vi "SwerveDrivePoseEst2_New.vi"(4 "VisionMeasurementStdDevs":T4=[[0.9], [0.9], [0.9]], 6 "StateStdDevs":T4=[[0.1], [0.1], [0.1]], 7 "SWERVE_DRIVE_KINEMATICS":T3 {"SavedModuleStates"."Angle"."SIN" format="%13.4f"; "SavedModuleStates"."Angle"."COS" format="%13.4f"; "SavedModuleStates"."Angle"."VALUE" format="%13.4f"; "PrevCoR"."Y" format="%14.3f"; "PrevCoR"."X" format="%14.3f"; "Modules"."Y" format="%14.3f"; "Modules"."X" format="%14.3f"}, 8 "InitialPose":T7={"TRANSLATION"={"X"=0.0, "Y"=0.0}, "ROTATION"={"VALUE"=0.0, "COS"=1.0, "SIN"=0.0}} {"ROTATION"."SIN" format="%13.4f"; "ROTATION"."COS" format="%13.4f"; "ROTATION"."VALUE" format="%13.4f"; "TRANSLATION"."Y" format="%14.3f"; "TRANSLATION"."X" format="%14.3f"}, 10 "Module Positions":T1[](array[typedef]) {"Angle"."SIN" format="%13.4f"; "Angle"."COS" format="%13.4f"; "Angle"."VALUE" format="%13.4f"}, 11 "gyroAngle":T2={"VALUE"=0.0, "COS"=1.0, "SIN"=0.0} {"SIN" format="%13.4f"; "COS" format="%13.4f"; "VALUE" format="%13.4f"}) -> (0 "Error":errorcluster, 3 "SwerveDrivePoseEstimate":T8={"M_Vision_K"=[], "m_nominal_dT"=0.0, "m_PrevTime_Sec"=0.0, "Pose_Buffer"={"TimeStamps"=[], "DataArray"=[], "Min_TimeStamp"=0.0, "Max_TimeStamp"=0.0, "ItemCount"=0, "MaxBufferTime"=0.0}, "Swerve_Drive_Kinematics"={"NumModules"=0, "InverseKinematics"=[], "ForwardKinematics"=[], "Modules"=[], "PrevCoR"={"X"=0.0, "Y"=0.0}, "SavedModuleStates"=[]}, "Swerve_Drive_Odom"={"POSE"={"TRANSLATION"={"X"=0.0, "Y"=0.0}, "ROTATION"={"VALUE"=0.0, "COS"=1.0, "SIN"=0.0}}, "GyroOffset"={"VALUE"=0.0, "COS"=1.0, "SIN"=0.0}, "PreviousAngle"={"VALUE"=0.0, "COS"=1.0, "SIN"=0.0}, "PrevModulePositions"=[], "NumModules"=0}, "M_Q"=[[0.0], [0.0], [0.0]], "NumModules"=-1} {"Swerve_Drive_Odom"."PrevModulePositions"."Angle"."SIN" format="%13.4f"; "Swerve_Drive_Odom"."PrevModulePositions"."Angle"."COS" format="%13.4f"; "Swerve_Drive_Odom"."PrevModulePositions"."Angle"."VALUE" format="%13.4f"; "Swerve_Drive_Odom"."PreviousAngle"."SIN" format="%13.4f"; "Swerve_Drive_Odom"."PreviousAngle"."COS" format="%13.4f"; "Swerve_Drive_Odom"."PreviousAngle"."VALUE" format="%13.4f"; "Swerve_Drive_Odom"."GyroOffset"."SIN" format="%13.4f"; "Swerve_Drive_Odom"."GyroOffset"."COS" format="%13.4f"; "Swerve_Drive_Odom"."GyroOffset"."VALUE" format="%13.4f"; "Swerve_Drive_Odom"."POSE"."ROTATION"."SIN" format="%13.4f"; "Swerve_Drive_Odom"."POSE"."ROTATION"."COS" format="%13.4f"; "Swerve_Drive_Odom"."POSE"."ROTATION"."VALUE" format="%13.4f"; "Swerve_Drive_Odom"."POSE"."TRANSLATION"."Y" format="%14.3f"; "Swerve_Drive_Odom"."POSE"."TRANSLATION"."X" format="%14.3f"; "Swerve_Drive_Kinematics"."SavedModuleStates"."Angle"."SIN" format="%13.4f"; "Swerve_Drive_Kinematics"."SavedModuleStates"."Angle"."COS" format="%13.4f"; "Swerve_Drive_Kinematics"."SavedModuleStates"."Angle"."VALUE" format="%13.4f"; "Swerve_Drive_Kinematics"."PrevCoR"."Y" format="%14.3f"; "Swerve_Drive_Kinematics"."PrevCoR"."X" format="%14.3f"; "Swerve_Drive_Kinematics"."Modules"."Y" format="%14.3f"; "Swerve_Drive_Kinematics"."Modules"."X" format="%14.3f"})   [LabVIEW 2019, in "Trajectory_Library.lvlib"]
doc: "This class wraps Swerve Drive Odometry to fuse latency-compensated vision measurements with differential drive encoder measurements. It is intended to be a drop-in replacement for SwerveDrvOdometry; in fact, if you never call SwerveDrvPoseEst2_AddVisionMeasurement and only call SwerveDrvPoseEst2_Update then this will behave exactly the same as SwerveDrvOdometry.\n \nSwerveDrvPoseEst2_Update should be called every robot loop.\n \nSwrveDrvPoseEst2_AddVisionMeasurement can be called as infrequently as you want. If you never call it then this set of VI will behave exactly like regular encoder odometry.\n\nConstructs a SwerveDrivePoseEstimator2.\n\nThe default standard deviations of the model states are 0.1 meters for x, 0.1 meters for y, and 0.1 radians for heading. The default standard deviations of the vision measurements are 0.9 meters for x, 0.9 meters for y, and 0.9 radians for heading.\n\nInputs: \n - kinematics -- SwerveDriveKinematics -- A correctly-configured kinematics data cluster for your drivetrain.\n - gyroAngle -- Rotation2d -- The current gyro angle.\n - ModulePositions -- ModulePositions -- The current module positions.\n - initialPoseMeters -- Pose2d -- The starting pose estimate.\n - stateStdDevs -- <3,1> matrix -- Standard deviations of the pose estimate (x position in meters, y position in meters, and heading in radians). Increase these numbers to trust your state estimate less.\n - visionMeasurementStdDevs -- <3,1> matrix -- Standard deviations of the vision pose measurement (x position in meters, y position in meters, and heading in radians). Increase these numbers to trust the vision pose measurement less.\n \nOutputs:\n -- SwerveDrivePoseEst2 -- SwerveDrivePoseEst2 -- Created data cluster."
uses:
  Trajectory_Library.lvlib
  <vilib>/Analysis/Matrix/Datatypes/RealMatrix.ctl
  <vilib>/Analysis/Matrix/NI_Matrix.lvlib
  TypeDef/TRANSLATION2D.ctl
  TypeDef/ROTATION2D.ctl
  TypeDef/POSE2D.ctl
  TypeDef/TIME_INTERPOLATABLE_VARIANT.ctl
  TypeDef/SWERVE_DRIVE_MODULE_STATE.ctl
  TypeDef/SWERVE_DRIVE_KINEMATICS.ctl
  TypeDef/SWERVE_DRIVE_MODULE_POSITION.ctl
  TypeDef/SWERVE_DRIVE_ODOMETRY.ctl
  TypeDef/SWERVE_DRIVE_POSE_EST2.ctl
panel:
  # "<3,1>"
  # "<3, 1>"
  # "<3, 1>"
  # "<3, 3>"
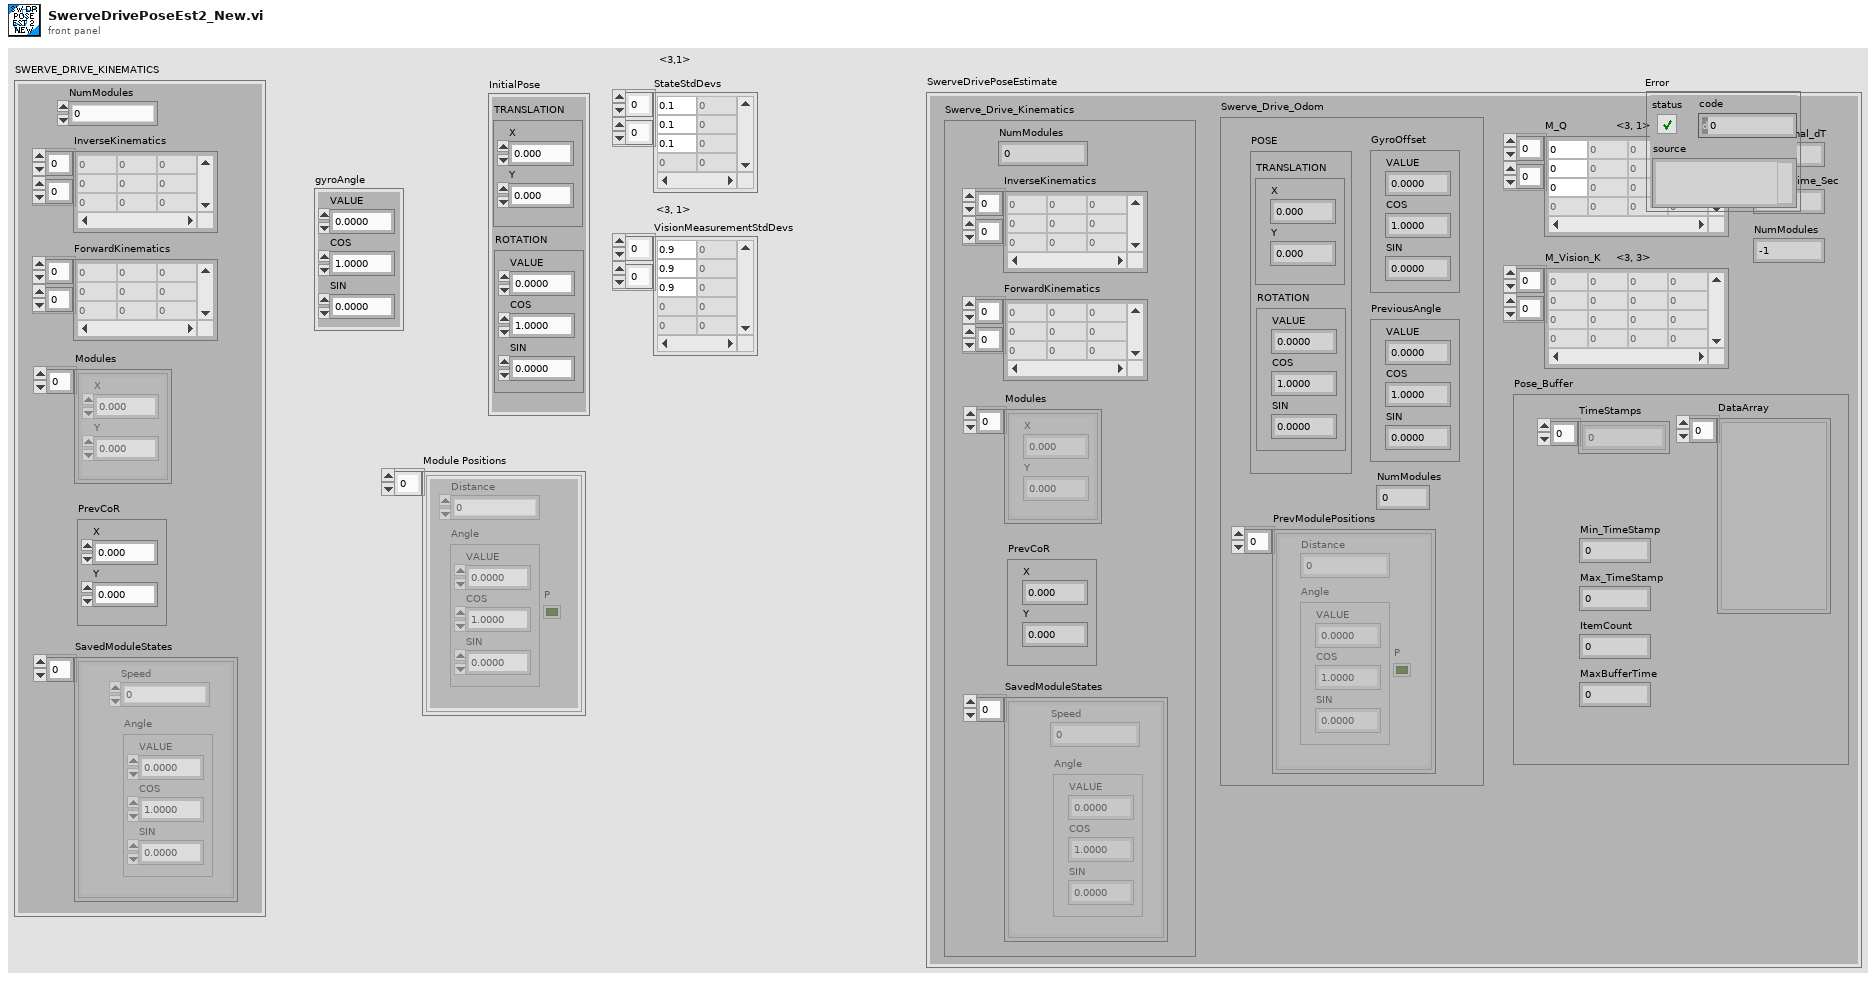
[diagram p1: front panel]
types:
  T1 = typedef "Trajectory_Library.lvlib/SWERVE_DRIVE_MODULE_POSITION.ctl" = cluster{"Distance":dbl, "Angle":T2, "P":bool}
  T2 = typedef "Trajectory_Library.lvlib/ROTATION2D.ctl" = cluster{"VALUE":dbl, "COS":dbl, "SIN":dbl}
  T3 = typedef "Trajectory_Library.lvlib/SWERVE_DRIVE_KINEMATICS.ctl" = cluster{"NumModules":i32, "InverseKinematics":T4, "ForwardKinematics":T4, "Modules":T5[], "PrevCoR":T5, "SavedModuleStates":T6[]}
  T4 = typedef "NI_Matrix.lvlib/RealMatrix.ctl" = dbl[][]
  T5 = typedef "Trajectory_Library.lvlib/TRANSLATION2D.ctl" = cluster{"X":dbl, "Y":dbl}
  T6 = typedef "Trajectory_Library.lvlib/SWERVE_DRIVE_MODULE_STATE.ctl" = cluster{"Speed":dbl, "Angle":T2}
  T7 = typedef "Trajectory_Library.lvlib/POSE2D.ctl" = cluster{"TRANSLATION":T5, "ROTATION":T2}
  T8 = typedef "Trajectory_Library.lvlib/SWERVE_DRIVE_POSE_EST2.ctl" = cluster{"M_Vision_K":T4, "m_nominal_dT":dbl, "m_PrevTime_Sec":dbl, "Pose_Buffer":T9, "Swerve_Drive_Kinematics":T3, "Swerve_Drive_Odom":T10, "M_Q":T4, "NumModules":i32}
  T9 = typedef "Trajectory_Library.lvlib/TIME_INTERPOLATABLE_VARIANT.ctl" = cluster{"TimeStamps":dbl[], "DataArray":variant[], "Min_TimeStamp":dbl, "Max_TimeStamp":dbl, "ItemCount":i32, "MaxBufferTime":dbl}
  T10 = typedef "Trajectory_Library.lvlib/SWERVE_DRIVE_ODOMETRY.ctl" = cluster{"POSE":T7, "GyroOffset":T2, "PreviousAngle":T2, "PrevModulePositions":T1[], "NumModules":i32}
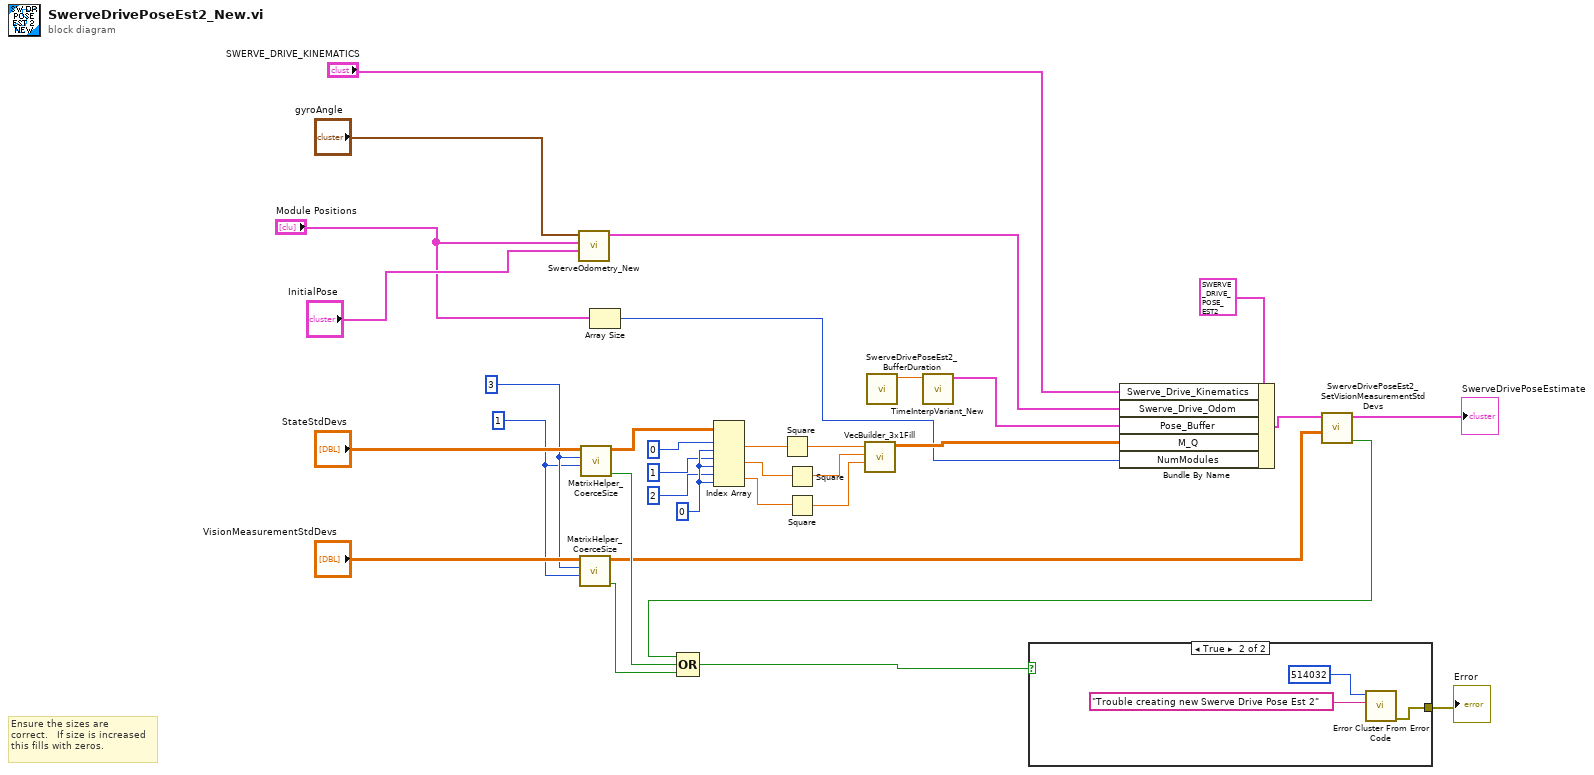
[diagram p0: block diagram]
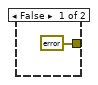
[diagram p2: hidden frame]
diagram:
  w19 = 0 ("index (col)")
  w22 = 1 ("Outputs")
  w23 = 3 ("States")
  # "Ensure the sizes are\ncorrect.   If size is increased \nthis fills with zeros."
  n1 = call "SwerveOdometry_New.vi"("InitialPose"="InitialPose", "Module Positions"="Module Positions", "gyroAngle"="gyroAngle") -> ("SWERVE_DRIVE_ODOMETRY"=w25:T10)  [unwired: 8 in]
  n2 = call "MatrixHelper_CoerceSize.vi"("Columns"=w22, "Rows"=w23, "input matrix"="VisionMeasurementStdDevs") -> ("Coerced"=w9:bool, "output matrix"=w6:T4)  [unwired: 7 in]
  n3 = call "MatrixHelper_CoerceSize.vi"("Columns"=w22, "Rows"=w23, "input matrix"="StateStdDevs") -> ("Coerced"=w31:bool, "output matrix"=w21:T4)  [unwired: 7 in]
  n4 = Array Size(array="Module Positions") -> (size(s)=w1:i32)
  n5 = Index Array(array=w21, index (row) #1=0 ("index (row)"), index (col) #1=w19, index (row) #2=1 ("index (row)"), index (col) #2=w19, index (row) #3=2 ("index (row)"), index (col) #3=w19) -> (element #1=w16:dbl, element #2=w15:dbl, element #3=w14:dbl)
  n6 = Square(x=w16) -> (x^2=w13:dbl)
  n7 = Square(x=w15) -> (x^2=w12:dbl)
  n8 = Square(x=w14) -> (x^2=w11:dbl)
  n9 = call "VecBuilder_3x1Fill.vi"("R2"=w11, "R1"=w12, "R0"=w13) -> ("output matrix"=w10:T4)  [unwired: 8 in]
  n10 = call "SwerveDrivePoseEst2_BufferDuration.vi"() -> ("Buffer Duration (Sec)"=w5:dbl)  [unwired: 11 in]
  n11 = call "TimeInterpVariant_New.vi"("MaxTime"=w5) -> ("TimeInterpVariant"=w24:T9)  [unwired: 10 in]
  n12 = Bundle By Name(cluster=T8 {"M_Vision_K"=[], "m_nominal_dT"=0.0, "m_PrevTime_Sec"=0.0, "Pose_Buffer"={"TimeStamps"=[], "DataArray"=[], "Min_TimeStamp"=0.0, "Max_TimeStamp"=0.0, "ItemCount"=0, "MaxBufferTime"=0.0}, "Swerve_Drive_Kinematics"={"NumModules"=0, "InverseKinematics"=[], "ForwardKinematics"=[], "Modules"=[], "PrevCoR"={"X"=0.0, "Y"=0.0}, "SavedModuleStates"=[]}, "Swerve_Drive_Odom"={"POSE"={"TRANSLATION"={"X"=0.0, "Y"=0.0}, "ROTATION"={"VALUE"=0.0, "COS"=1.0, "SIN"=0.0}}, "GyroOffset"={"VALUE"=0.0, "COS"=1.0, "SIN"=0.0}, "PreviousAngle"={"VALUE"=0.0, "COS"=1.0, "SIN"=0.0}, "PrevModulePositions"=[], "NumModules"=0}, "M_Q"=[[0.0], [0.0], [0.0]], "NumModules"=-1} ("DiffDrivePoseEstimate 2"), "Swerve_Drive_Kinematics"="SWERVE_DRIVE_KINEMATICS", "Swerve_Drive_Odom"=w25, "Pose_Buffer"=w24, "M_Q"=w10, "NumModules"=w1) -> (w4:T8)
  n13 = call "SwerveDrivePoseEst2_SetVisionMeasurementStdDevs.vi"("VisionMeasurementStdDevs"=w6, "in SwerveDrivePoseEstimate2"=w4) -> ("Size Coerced"=w7:bool, "Out SwerveDrivePoseEstimate2"=→"SwerveDrivePoseEstimate":T8)  [unwired: 8 in]
  n14 = Compound Arithmetic op=OR(w7, w31, w9) -> (w8:bool)
  n15 = case shown="True" w8 {
    tunnel: [errorcluster {"status"=FALSE, "code"=0, "source"=""} ("error out") w37] -> w30
    frame False {
    }
    frame True {
      n16 = call <vilib>:"Error Cluster From Error Code.vi"("error message (\"\")"="Trouble creating new Swerve Drive Pose Est 2" ("error message (\"\")"), "error code (0)"=514032) -> ("error out"=w37:errorcluster)  [unwired: 7 in]
    }
  }
  "Error" <- w30
